vi "Pre-Arm.vi"(8 "error in (no error)":errorcluster, 11 "RP I-V Driver in":refnum<class "RP I-V Driver.lvclass">) -> (0 "error out":errorcluster, 3 "RP I-V Driver out":refnum<class "RP I-V Driver.lvclass">)   [LabVIEW 2024, in "RP I-V Driver.lvclass"]
uses:
  RP I-V Driver.lvclass
  Red Pitaya Digitizer/Red Pitaya Digitizer.lvclass
  RP I-V Driver.lvclass/RP I-V Driver.ctl
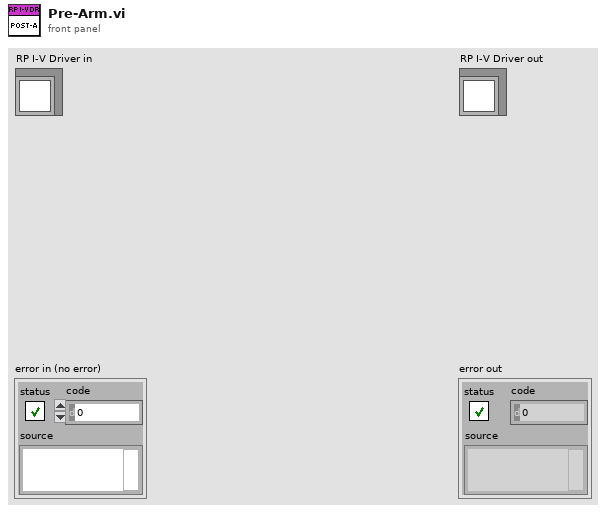
[diagram p1: front panel]
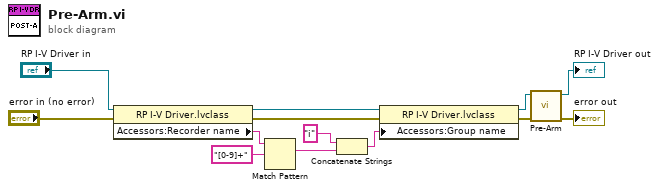
[diagram p0: block diagram]
diagram:
  n1 = property class="RP I-V Driver.lvclass"(reference="RP I-V Driver in", error in="error in (no error)") -> (reference out=w11:refnum<class "RP I-V Driver.lvclass">, error out=w10:errorcluster, "Accessors:Recorder name"=w12:string)
  n2 = Match Pattern(string=w12, regular expression="[0-9]+") -> (match substring=w8:string)  [unwired: 1 in, 3 out]
  n3 = Concatenate Strings("i", w8) -> (w7:string)
  n4 = property class="RP I-V Driver.lvclass"(reference=w11, error in=w10, "Accessors:Group name"=w7) -> (reference out=w4:refnum<class "RP I-V Driver.lvclass">, error out=w3:errorcluster)
  n5 = call-parent "Pre-Arm.vi"("error in (no error)"=w3, "Red Pitaya Digitizer in"=w4) -> ("error out"=→"error out":errorcluster, "Red Pitaya Digitizer out"=→"RP I-V Driver out":refnum<class "RP I-V Driver.lvclass">)  [unwired: 8 in]
